vi "SetTo0.vi"(10 "Longueur d'onde":dbl) -> (2 "Température 0":dbl)   [LabVIEW 2018]
uses:
  <vilib>/Analysis/NI_AALBase.lvlib
  <vilib>/Analysis/baseanly.llb/Mean (DBL).vi
  <vilib>/DAQmx/create/channels.llb/DAQmx Create Channel (DO-Digital Output).vi
  <vilib>/DAQmx/write.llb/DAQmx Write (Digital 1D Bool NChan 1Samp 1Line).vi
  <resource>/objmgr/daqmx.rc
  <vilib>/DAQmx/read.llb/DAQmx Read (Analog 1D Wfm NChan NSamp).vi
  <vilib>/DAQmx/configure/timing.llb/DAQmx Timing (Sample Clock).vi
  <vilib>/DAQmx/create/channels.llb/DAQmx Create Channel (AI-Voltage-Basic).vi
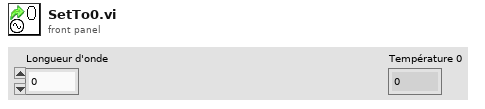
[diagram p1: front panel]
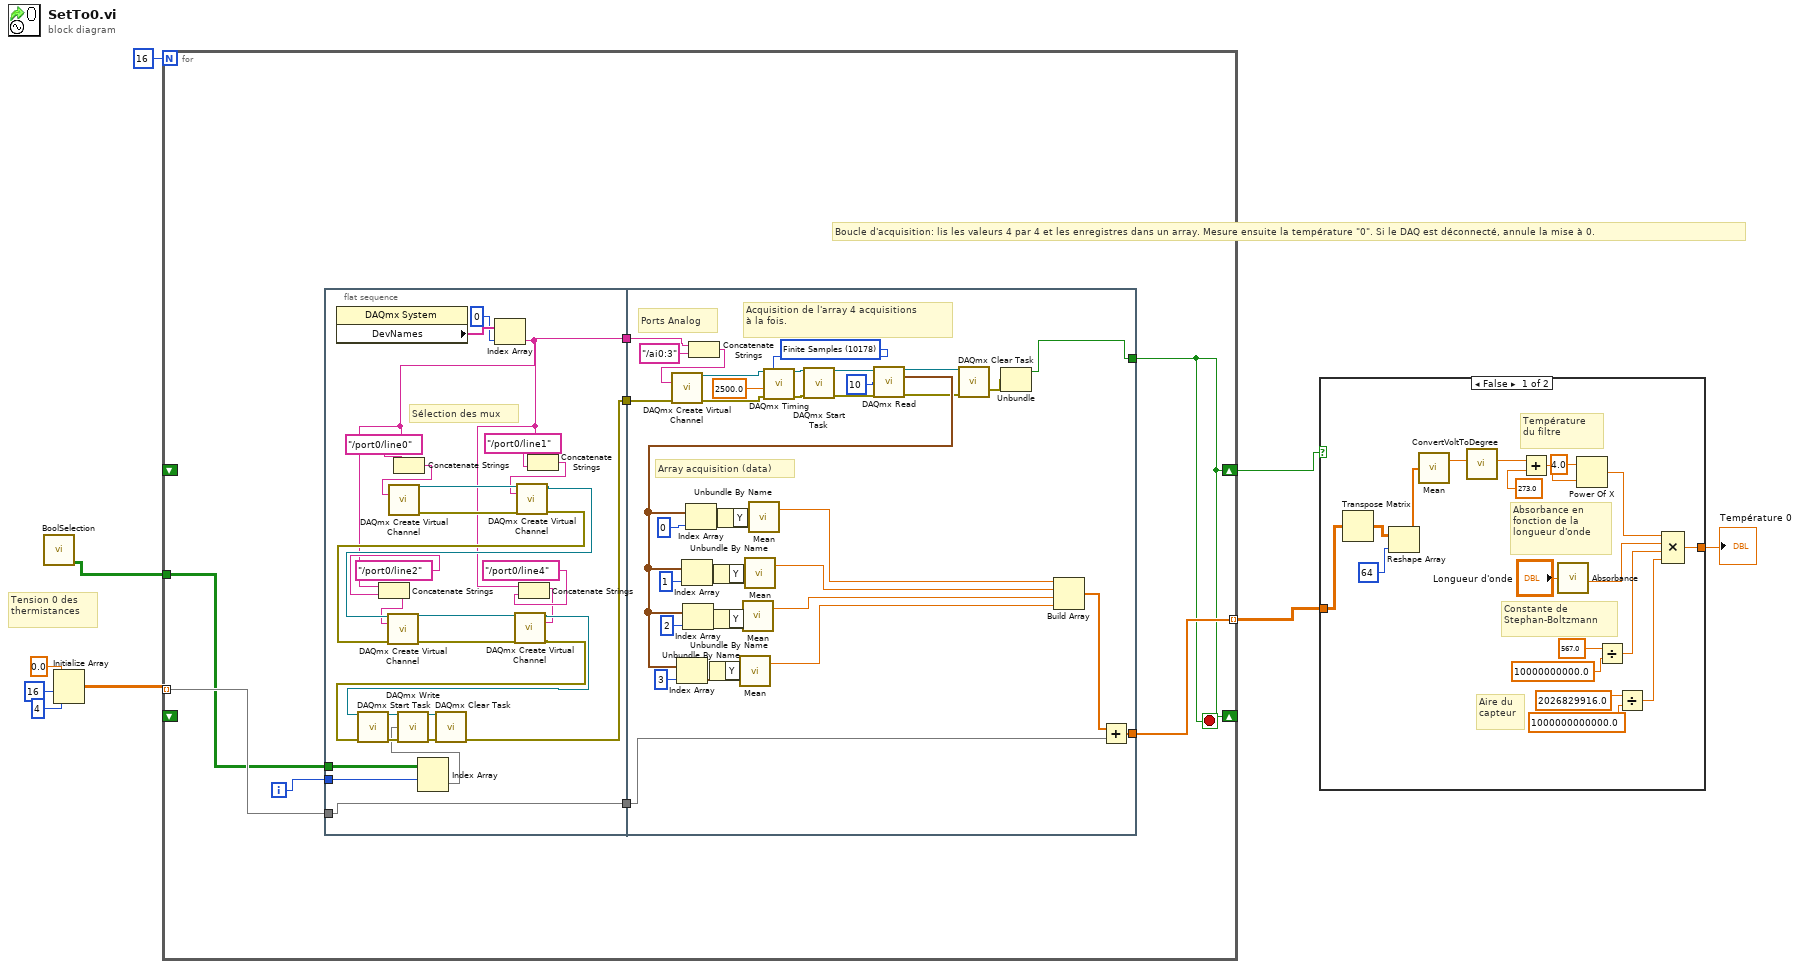
[diagram p0: block diagram]
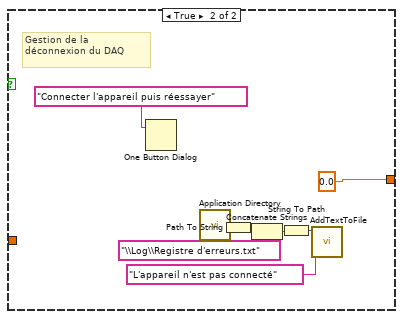
[diagram p2: hidden frame]
diagram:
  # "Tension 0 des \nthermistances"
  # "Boucle d'acquisition: lis les valeurs 4 par 4 et les enregistres dans un array. Mesure ensuite la température \"0\". Si le DAQ est déconnecté, annule la mise à 0."
  n1 = call "BoolSelection.vi"() -> ("BoolSelection"=w1:bool[][])  [unwired: 11 in]
  n2 = Initialize Array(0.0 ("element"), 16 ("dimension size"), 4 ("dimension size")) -> (w2:dbl[][])
  n3 = for {
    N: 16 -> [_]
    tunnel: w1 -> [w12]
    tunnel: w2 -> [w17] mode=indexing
    tunnel: [w11] -> w7 mode=indexing
    shift-right: [w10] -> _
    shift-left: _ -> [_]
    shift-right: [w10] -> w8
    shift-left: _ -> [_]
    i -> [w13]
    stop <- w10 stop-if-true
    n4 = flat-sequence {
      tunnel: w13 -> [w31]
      tunnel: [w42] -> w16
      tunnel: w12 -> [w30]
      tunnel: [w18] -> w15
      tunnel: [w19] -> w14
      tunnel: w17 -> [w18]
      tunnel: w16 -> [w74]
      tunnel: w15 -> [w54]
      tunnel: [w56] -> w11
      tunnel: w14 -> [w51]
      tunnel: [w46] -> w10
      frame #0 {
        # "Sélection des mux"
        n5 = property class="DAQmx System"() -> ("DevNames"=w29:tag[])  [unwired: 2 in, 2 out]
        n6 = Index Array(array=w30, index (row)=w31) -> (element=w43:bool[])  [unwired: 1 in]
        n7 = Index Array(array=w29, index=0) -> (element=w19:tag)
        n8 = Concatenate Strings(w19, "/port0/line2" ("string")) -> (w22:string)
        n9 = Concatenate Strings(w19, "/port0/line0" ("string")) -> (w27:string)
        n10 = call-poly <vilib>:"DAQmx Create Virtual Channel.vi"("lines"=w27) -> ("task out"=w38:refnum<k21>, "error out"=w39:errorcluster)  [unwired: 13 in]
        n11 = Concatenate Strings(w19, "/port0/line4" ("string")) -> (w20:string)
        n12 = Concatenate Strings(w19, "/port0/line1" ("string")) -> (w24:string)
        n13 = call-poly <vilib>:"DAQmx Create Virtual Channel.vi"("task in"=w38, "lines"=w24, "error in"=w39) -> ("task out"=w37:refnum<k21>, "error out"=w36:errorcluster)  [unwired: 11 in]
        n14 = call-poly <vilib>:"DAQmx Create Virtual Channel.vi"("task in"=w37, "lines"=w22, "error in"=w36) -> ("task out"=w34:refnum<k21>, "error out"=w35:errorcluster)  [unwired: 11 in]
        n15 = call-poly <vilib>:"DAQmx Create Virtual Channel.vi"("task in"=w34, "lines"=w20, "error in"=w35) -> ("task out"=w33:refnum<k21>, "error out"=w32:errorcluster)  [unwired: 11 in]
        n16 = call <vilib>:"DAQmx Start Task.vi"("task/channels in"=w33, "error in"=w32) -> ("task out"=w44:refnum<k21>, "error out"=w45:errorcluster)  [unwired: 12 in]
        n17 = call-poly <vilib>:"DAQmx Write.vi"("task/channels in"=w44, "data"=w43, "error in"=w45) -> ("task out"=w41:refnum<k21>, "error out"=w40:errorcluster)  [unwired: 10 in, 1 out]
        n18 = call <vilib>:"DAQmx Clear Task.vi"("task in"=w41, "error in"=w40) -> ("error out"=w42:errorcluster)  [unwired: 13 in]
      }
      frame #1 {
        w76 = 10178 items=["Finite Samples"=10178, "Continuous Samples"=10123, "Hardware Timed Single Point"=12522] ("sample mode")
        # "Ports Analog"
        # "Array acquisition (data)"
        # "Acquisition de l'array 4 acquisitions\nà la fois."
        n19 = Concatenate Strings(w51, "/ai0:3" ("string")) -> (w52:string)
        n20 = call-poly <vilib>:"DAQmx Create Virtual Channel.vi"("physical channels"=w52, "error in"=w74) -> ("task out"=w81:refnum<k21>, "error out"=w80:errorcluster)  [unwired: 12 in]
        n21 = call-poly <vilib>:"DAQmx Timing.vi"("task/channels in"=w81, "sample mode"=w76, "rate"=2500.0, "error in"=w80) -> ("task out"=w77:refnum<k21>, "error out"=w78:errorcluster)  [unwired: 10 in]
        n22 = call <vilib>:"DAQmx Start Task.vi"("task/channels in"=w77, "error in"=w78) -> ("task out"=w79:refnum<k21>, "error out"=w82:errorcluster)  [unwired: 12 in]
        n23 = call-poly <vilib>:"DAQmx Read.vi"("task/channels in"=w79, "number of samples per channel"=10, "error in"=w82) -> ("task out"=w58:refnum<k21>, "data"=w67:waveform(dbl)[], "error out"=w57:errorcluster)  [unwired: 10 in]
        n24 = Index Array(array=w67, index=3) -> (element=w63:waveform(dbl))
        n25 = Index Array(array=w67, index=1) -> (element=w65:waveform(dbl))
        n26 = Index Array(array=w67, index=2) -> (element=w64:waveform(dbl))
        n27 = Index Array(array=w67, index=0) -> (element=w66:waveform(dbl))
        n28 = Unbundle By Name(w63) -> ("Y"=w59:dbl[])
        n29 = Unbundle By Name(w65) -> ("Y"=w61:dbl[])
        n30 = Unbundle By Name(w64) -> ("Y"=w60:dbl[])
        n31 = Unbundle By Name(w66) -> ("Y"=w62:dbl[])
        n32 = call-poly <vilib>:"Mean.vi"("X"=w59) -> ("mean"=w47:dbl)  [unwired: 1 out]
        n33 = call-poly <vilib>:"Mean.vi"("X"=w60) -> ("mean"=w48:dbl)  [unwired: 1 out]
        n34 = call-poly <vilib>:"Mean.vi"("X"=w61) -> ("mean"=w49:dbl)  [unwired: 1 out]
        n35 = call-poly <vilib>:"Mean.vi"("X"=w62) -> ("mean"=w50:dbl)  [unwired: 1 out]
        n36 = call <vilib>:"DAQmx Clear Task.vi"("task in"=w58, "error in"=w57) -> ("error out"=w72:errorcluster)  [unwired: 13 in]
        n37 = Unbundle(w72) -> ("status"=w46:bool)  [unwired: 2 out]
        n38 = Build Array(w50, w49, w48, w47) -> (w55:dbl[])
        n39 = Add(x=w55, y=w54) -> (x+y=w56:dbl[])
      }
    }
  }
  n40 = case shown="False" w8 {
    tunnel: w7 -> [w87 _]
    tunnel: [w83 0.0] -> w9
    frame False {
      # "Constante de \nStephan-Boltzmann"
      # "Absorbance en\nfonction de la \nlongueur d'onde"
      # "Température \ndu filtre"
      # "Aire du\ncapteur"
      n41 = Transpose Matrix(1:w87) -> (0:w88:dbl[][])
      n42 = Reshape Array(w88, 64 ("dimension size")) -> (w85:dbl[])
      n43 = call-poly <vilib>:"Mean.vi"("X"=w85) -> ("mean"=w84:dbl)  [unwired: 1 out]
      n44 = call "ConvertVoltToDegree.vi"("Tension"=w84) -> ("Température"=w93:dbl)  [unwired: 10 in]
      n45 = Add(x=w93, y=273.0) -> (x+y=w100:dbl)
      n46 = call "Absorbance.vi"("Longueur d'onde"="Longueur d'onde") -> ("absorbance"=w90:dbl)  [unwired: 10 in]
      n47 = Power Of X(1:w100, 2:4.0 ("y")) -> (0:w89:dbl)
      n48 = Divide(x=567.0, y=10000000000.0) -> (x/y=w91:dbl)
      n49 = Divide(x=2026829916.0, y=1000000000000.0) -> (x/y=w92:dbl)
      n50 = Compound Arithmetic op=MULTIPLY(w89, w90, w91, w92) -> (w83:dbl)
    }
    frame True {
      # "Gestion de la \ndéconnexion du DAQ"
      n51 = One Button Dialog(message="Connecter l'appareil puis réessayer") -> ()  [unwired: 1 in, 1 out]
      n52 = call <vilib>:"Application Directory.vi"() -> ("Application Directory"=w105:path)
      n53 = Path To String(path=w105) -> (string=w106:string)
      n54 = Concatenate Strings(w106, "\\Log\\Registre d'erreurs.txt") -> (w107:string)
      n55 = String To Path(string=w107) -> (path=w103:path)
      n56 = call "AddTextToFile.vi"("Ajouter du texte"="L'appareil n'est pas connecté", "Fichier"=w103) -> ()  [unwired: 10 in]
    }
  }
  "Température 0" <- w9
